vi "New JSON (Value[]).vi"(8 "error in (no error)":errorcluster, 10 "JSON Datatypes":refnum<class "JSON Value.lvclass">[](array[class])) -> (0 "error out":errorcluster, 3 "JSON Value out":refnum<class "JSON Value.lvclass">)   [LabVIEW 2016, in "JSON Value.lvclass"]
doc: "Creates a new JSON Array initialized with JSON Boolean objects of the values specified by JSON Datatypes"
uses:
  JSON Value.lvclass
  JSON Value.lvclass/JSON Value.ctl
  JSON Types.ctl
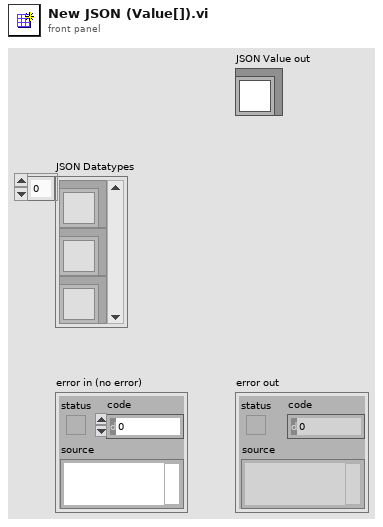
[diagram p1: front panel]
types:
  T1 = typedef "JSON Value.lvclass/JSON Types.ctl" = enum8{"String", "Numeric", "Boolean", "NULL", "Object", "Array"}
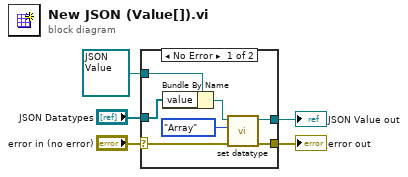
[diagram p0: block diagram]
diagram:
  n1 = case shown="No Error" "error in (no error)" {
    selector: "error in (no error)" -> [w11 w14]
    tunnel: [w9 w14] -> w4
    tunnel: [w7 w13] -> w3
    tunnel: refnum<class "JSON Value.lvclass"> refnum ("JSON out") -> [w12 w13]
    tunnel: "JSON Datatypes" -> [w10 _]
    frame No Error {
      n2 = Bundle By Name(cluster=w12, "value"=w10) -> (w8:refnum<class "JSON Value.lvclass">)
      n3 = call "set datatype.vi"("error in (no error)"=w11, "datatype"=JSON_Types."Array", "JSON Helper in"=w8) -> ("error out"=w9:errorcluster, "JSON Helper out"=w7:refnum<class "JSON Value.lvclass">)  [unwired: 7 in]
    }
    frame Error {
    }
  }
  "error out" <- w4
  "JSON Value out" <- w3
